vi "PH_Stepmotor_BaseClass.PC Write Axis PSDB.vi"(0 "i ref in":refnum<vi>, 5 "error IO":errorcluster) -> (14 "i ref out":refnum<vi>, 19 "error out":errorcluster)   [LabVIEW 2014, in "PH_Stepmotor_BaseClass.lvlib"]
doc: "This is the proc case which writes axis data to the PHELIX shot data base."
uses:
  PH_Stepmotor_BaseClass.lvlib
  PH_Stepmotor_BaseClass.Motor Type.ctl
  PH_PSDBWriter/PH_PSDBWriter.PSDB Dataset.ctl
  PH_PSDBWriter/PH_PSDBWriter.2D dataset.ctl
  CSlibraries-extern/psdb_lv/PSDB_AxisDescription.ctl
  PH_PSDBWriter/PH_PSDBWriter.Boolean dataset.ctl
  PH_PSDBWriter/PH_PSDBWriter.Image dataset.ctl
  <vilib>/vision/Image Controls.llb/IMAQ Image.ctl
  PH_PSDBWriter/PH_PSDBWriter.Numeric dataset.ctl
  PH_PSDBWriter/PH_PSDBWriter.String dataset.ctl
  PH_PSDBWriter/PH_PSDBWriter.Data Status.ctl
  PH_PSDBWriter/PH_PSDBWriter.lvlib
  CS_Core/CSSystem/CSSystemLib/CSSystemLib.lvlib
  CSlibraries-extern/psdb_lv/PSDB.lvlib
panel:
  in  "SW Scale.Motor Type":T1
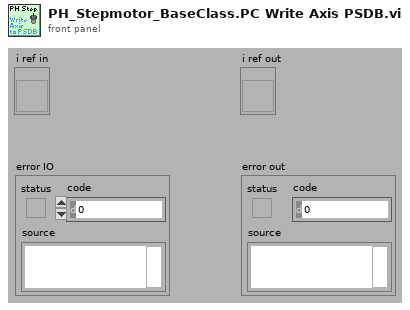
[diagram p1: front panel]
types:
  T1 = typedef "PH_Stepmotor_BaseClass.lvlib/PH_Stepmotor_BaseClass.Motor Type.ctl" = enum16{"Unspecific", "OWIS 49.120.2633", "OWIS 49.060.1033", "OWIS 43.040.2558", "Diamond Motion 2200 series", "OWIS 49.120.266B.MV6", "Calorimeter", "Linear Stage 1", "MICOS VT-80", "MICOS VT-80 S", "Standa Rotstage nt0.95A", "PUF RA 320.200", "PUF RA 800.200", "PUF RA 800.400", "PUF RA 400.50", "1324.nn.800.50", "1324.n9c.800.50", "1324.nn.320.200", "1324.nn.400.200", "1324.nn.800.200", "1324.nn.400.50", "1324.8c9c.800.50", "1324.8c9c.400.200"}
  T2 = typedef "PH_PSDBWriter.lvlib/PH_PSDBWriter.PSDB Dataset.ctl" = cluster{"Version":i32, "2D data Input":T3[], "Boolean Input":T5[], "Image Input":T6[], "Numeric Input":T8[], "String Input":T9[]}
  T3 = typedef "PH_PSDBWriter.lvlib/PH_PSDBWriter.2D dataset.ctl" = cluster{"name":string, "data":dbl[][], "axis description":T4}
  T4 = typedef "PSDB.lvlib/PSDB_AxisDescription.ctl" = cluster{"x axis label":string, "y axis label":string, "x axis unit":string, "y axis unit":string}
  T5 = typedef "PH_PSDBWriter.lvlib/PH_PSDBWriter.Boolean dataset.ctl" = cluster{"name":string, "data":bool, "unit":string}
  T6 = typedef "PH_PSDBWriter.lvlib/PH_PSDBWriter.Image dataset.ctl" = cluster{"name":string, "data":T7, "unit":string}
  T7 = typedef "IMAQ Image.ctl" = refnum<image>
  T8 = typedef "PH_PSDBWriter.lvlib/PH_PSDBWriter.Numeric dataset.ctl" = cluster{"name":string, "data":dbl, "unit":string}
  T9 = typedef "PH_PSDBWriter.lvlib/PH_PSDBWriter.String dataset.ctl" = cluster{"name":string, "data":string, "unit":string}
  T10 = typedef "PH_Stepmotor_BaseClass.lvlib/PH_Stepmotor_BaseClass.i attribute.ctl" = cluster{"Device Error":errorcluster, "Axes PSDB Thread":cluster{"Ref":refnum<vi>, "Q-Ref":refnum<queue>, "Data Status":T11}, "Axes":T12[], "Axes PSDB Infos":cluster{"GUI Name":string, "PSDB Instance ID":i32, "PSDB Status Service ID":i32, "Axis":i32, "Class":string}[], "GUI Refs":T16}
  T11 = typedef "PH_PSDBWriter.lvlib/PH_PSDBWriter.Data Status.ctl" = i16
  T12 = typedef "PH_Stepmotor_BaseClass.lvlib/PH_Stepmotor_BaseClass.Axis Attributes.ctl" = cluster{"Settings":T13, "Endswitch?":bool, "DIM Service IDs":T14, "Activity":T15, "Configured?":bool, "Position":cluster{"Current":i32, "Target":i32}, "Position to set":cluster{"New?":bool, "Wanted":i32}, "Stop?":bool, "Reset?":bool, "Move?":bool, "Nothing connected?":bool}
  T13 = typedef "PH_Stepmotor_BaseClass.lvlib/PH_Stepmotor_BaseClass.Axis Settings.ctl" = cluster{"Sign change":bool, "Width":dbl, "Calibration":dbl, "Unit":string, "Motor Type":T1, "Unit Width":string, "Unit CF":string}
  T14 = typedef "PH_Stepmotor_BaseClass.lvlib/PH_Stepmotor_BaseClass.Axis DIM Service IDs.ctl" = cluster{"Settings":i32, "Information":i32}
  T15 = typedef "PH_Stepmotor_BaseClass.lvlib/PH_Stepmotor_BaseClass.Axis Activity.ctl" = enum16{"No Information", "stopped", "running", "Failure", "Alarm", "stopped at backward ES", "stopped at foreward ES"}
  T16 = typedef "PH_Stepmotor_BaseClass.lvlib/PH_Stepmotor_BaseClass.GUI Refs.ctl" = cluster{"Axes Configuration":refnum<vi>, "Device Error":refnum<vi>, "Axes PSDB Infos":refnum<vi>}
  T17 = cluster{"GUI Name":string, "PSDB Instance ID":i32, "PSDB Status Service ID":i32, "Axis":i32, "Class":string}[]
  T18 = typedef "PH_PSDBWriter.lvlib/PH_PSDBWriter.i attribute.ctl" = cluster{"PSDB Status Service ID":i32, "Instance ID":i32, "Shot #":i32, "Subsystem":T19, "Data Status":T11, "Ref PSDB Status":refnum<vi>, "PSDB Error Code":i32, "PSDB Dataset":T2, "PSDB Thread":cluster{"Ref":refnum<vi>, "Q-Ref":refnum<queue>}, "PSDB Credentials":T20}
  T19 = typedef "PH_PSDBWriter.lvlib/PH_PSDBWriter.PHELIX-Subsystems.ctl" = i32
  T20 = typedef "PH_Common.lvlib/PH_Connection.PSDB Credentials.ctl" = cluster{"PW":string, "ID":string, "DS":string}
  T21 = cluster{"PSDB Instance ID":i32, "PSDB Dataset":T2}
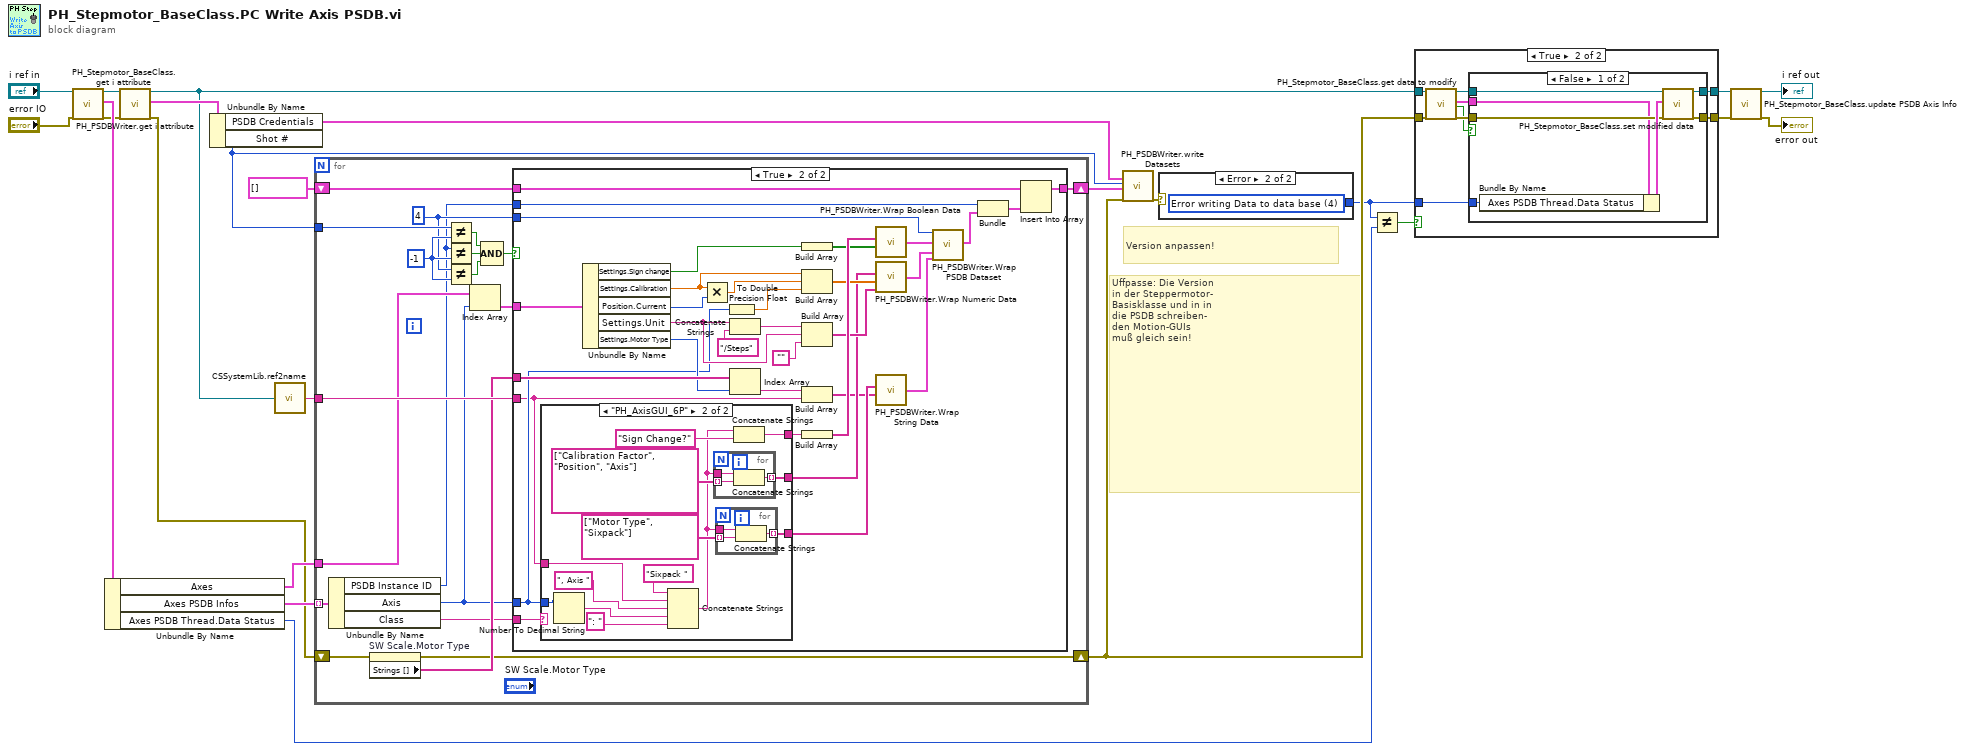
[diagram p0: block diagram]
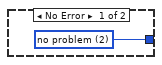
[diagram p4: hidden frame]
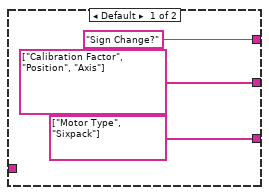
[diagram p6: hidden frame]
diagram:
  # "Uffpasse: Die Version\nin der Steppermotor-\nBasisklasse und in in\ndie PSDB schreiben-\nden Motion-GUIs\nmuß gleich sein!"
  # "Version anpassen!"
  n1 = call "PH_Stepmotor_BaseClass.get i attribute.vi"("i ref in"="i ref in", "error in (no error)"="error IO") -> ("i ref out"=w11:refnum<vi>, "i attribute"=w12:T10, "error out"=w9:errorcluster)  [unwired: 15 in]
  n2 = Unbundle By Name(w12) -> ("Axes"=w19:T12[], "Axes PSDB Infos"=w20:T17, "Axes PSDB Thread.Data Status"=w4:T11)
  n3 = call "PH_PSDBWriter.get i attribute.vi"("i ref in"=w11, "error in (no error)"=w9) -> ("i ref out"=w6:refnum<vi>, "i attribute"=w13:T18, "error out"=w5:errorcluster)  [unwired: 15 in]
  n4 = Unbundle By Name(w13) -> ("PSDB Credentials"=w1:T20, "Shot #"=w14:i32)
  n5 = call "CSSystemLib.ref2name.vi"("obj refnum"=w6) -> ("name"=w18:string)
  n6 = for {
    tunnel: w20 -> [w28] mode=indexing
    tunnel: w19 -> [w35]
    tunnel: w18 -> [w43]
    shift-right: [w32] -> w8
    shift-left: w5 -> [w33]
    tunnel: w14 -> [w40]
    shift-right: [w27] -> w15
    shift-left: cluster{"Version":i32, "PSDB Dataset":T2}[] [] ("Array") -> [w26]
    w29 = 4 ("Version")
    w42 = -1 ("y")
    n7 = Unbundle By Name(w28) -> ("PSDB Instance ID"=w25:i32, "Axis"=w30:i32, "Class"=w31:string)
    n8 = property on="SW Scale.Motor Type" class="Enum (strict)"(error in=w33) -> (error out=w32:errorcluster, "Strings []"=w36:string[])  [unwired: 1 in, 1 out]
    n9 = Not Equal?(x=w40, y=w42) -> (x != y?=w41:bool)
    n10 = Not Equal?(x=w25, y=w42) -> (x != y?=w39:bool)
    n11 = Not Equal?(x=w29, y=w42) -> (x != y?=w38:bool)
    n12 = Index Array(array=w35, index=w30) -> (element=w34:T12)
    n13 = Compound Arithmetic op=AND(w41, w39, w38) -> (w37:bool)
    n14 = case shown="True" w37 {
      tunnel: w36 -> [_ w77]
      tunnel: w43 -> [_ w66]
      tunnel: w29 -> [_ w49]
      tunnel: w34 -> [_ w71]
      tunnel: w31 -> [_ w69]
      tunnel: w30 -> [_ w67]
      tunnel: [w44 w47] -> w27
      tunnel: w26 -> [w44 w46]
      tunnel: w25 -> [_ w45]
      frame False {
      }
      frame True {
        n15 = case shown="\"PH_AxisGUI_6P\"" w69 {
          tunnel: w67 -> [_ w92]
          tunnel: [string[] ["Calibration Factor", "Position", "Axis"] w89] -> w56
          tunnel: ["Sign Change?" w88] -> w62
          tunnel: [string[] ["Motor Type", "Sixpack"] w84] -> w55
          tunnel: w66 -> [_ w82]
          frame Default {
          }
          frame "PH_AxisGUI_6P" {
            n16 = Number To Decimal String(number=w92) -> (decimal integer string=w91:string)  [unwired: 1 in]
            n17 = Concatenate Strings("Sixpack " ("string"), w82, ", Axis ", w91, ": " ("string")) -> (w85:string)
            n18 = for {
              tunnel: [w99] -> w89 mode=indexing
              tunnel: string[] ["Calibration Factor", "Position", "Axis"] -> [w98] mode=indexing
              tunnel: w85 -> [w97]
              n19 = Concatenate Strings(w97, w98) -> (w99:string)
            }
            n20 = for {
              tunnel: [w96] -> w84 mode=indexing
              tunnel: string[] ["Motor Type", "Sixpack"] -> [w95] mode=indexing
              tunnel: w85 -> [w94]
              n21 = Concatenate Strings(w94, w95) -> (w96:string)
            }
            n22 = Concatenate Strings(w85, "Sign Change?") -> (w88:string)
          }
        }
        n23 = Unbundle By Name(w71) -> ("Settings.Sign change"=w60:bool, "Settings.Calibration"=w65:dbl, "Position.Current"=w64:i32, "Settings.Unit"=w72:string, "Settings.Motor Type"=w76:T1)
        n24 = Multiply(x=w65, y=w64) -> (x*y=w63:dbl)
        n25 = To Double Precision Float(number=w67) -> (double precision float=w68:dbl)
        n26 = Concatenate Strings(w72, "/Steps" ("string")) -> (w74:string)
        n27 = Index Array(array=w77, index=w76) -> (element=w73:string)
        n28 = Build Array(w60) -> (w59:bool[])
        n29 = Build Array(w65, w63, w68) -> (w57:dbl[])
        n30 = Build Array(w74, w72, "" ("element")) -> (w58:string[])
        n31 = Build Array(w73, w66) -> (w54:string[])
        n32 = Build Array(w62) -> (w61:string[])
        n33 = call "PH_PSDBWriter.Wrap Boolean Data.vi"("Data Array"=w59, "Name Array"=w61) -> ("PSDB Boolean Data Array"=w53:T5[])  [unwired: 2 in]
        n34 = call "PH_PSDBWriter.Wrap Numeric Data.vi"("Unit Array"=w58, "Data Array"=w57, "Name Array"=w56) -> ("PSDB Numeric Data Array"=w52:T8[])  [unwired: 1 in]
        n35 = call "PH_PSDBWriter.Wrap String Data.vi"("Data Array"=w54, "Name Array"=w55) -> ("PSDB String Data Array"=w51:T9[])  [unwired: 2 in]
        n36 = call "PH_PSDBWriter.Wrap PSDB Dataset.vi"("Version"=w49, "Boolean Input"=w53, "Numeric Input"=w52, "String Input"=w51) -> ("PSDB Dataset"=w50:T2)  [unwired: 15 in]
        n37 = Bundle("PSDB Instance ID"=w45, "PSDB Dataset"=w50) -> (w48:T21)  [unwired: 1 in]
        n38 = Insert Into Array(array=w46, new element=w48) -> (w47:cluster{"Version":i32, "PSDB Dataset":T2}[])  [unwired: 1 in]
      }
    }
  }
  n39 = call "PH_PSDBWriter.write Datasets.vi"("PSDB Credentials"=w1, "Shot #"=w14, "Datasets"=w15, "error in (no error)"=w8) -> ("error out"=w17:errorcluster)  [unwired: 15 in]
  n40 = case shown="Error" w17 {
    tunnel: [w100 w101] -> w3
    frame No Error {
      w100 = T11 2 items=["no info", "no Data collection", "no problem", "Error getting the instance ID", "Error writing Data to data base", "Error concerning the subsystem"] ("Data Status")
    }
    frame Error {
      w101 = T11 4 items=["no info", "no Data collection", "no problem", "Error getting the instance ID", "Error writing Data to data base", "Error concerning the subsystem"] ("Data Status")
    }
  }
  n41 = Not Equal?(x=w3, y=w4) -> (x != y?=w2:bool)
  n42 = case shown="True" w2 {
    tunnel: [w103 w112] -> w23
    tunnel: [w102 w111] -> w21
    tunnel: w8 -> [w102 w106]
    tunnel: w6 -> [w103 w105]
    tunnel: w3 -> [_ w104]
    frame False {
    }
    frame True {
      n43 = call "PH_Stepmotor_BaseClass.get data to modify.vi"("i ref in"=w105, "error in (no error)"=w106) -> ("i ref out"=w110:refnum<vi>, "i attribute"=w108:T10, "timed out"=w107:bool, "error out"=w109:errorcluster)  [unwired: 14 in]
      n44 = case shown="False" w107 {
        tunnel: [w119 w121] -> w112
        tunnel: [w118 w120] -> w111
        tunnel: w110 -> [w116 w121]
        tunnel: w109 -> [w115 w120]
        tunnel: w108 -> [w114 _]
        tunnel: w104 -> [w113 _]
        frame False {
          n45 = Bundle By Name(cluster=w114, "Axes PSDB Thread.Data Status"=w113) -> (w117:T10)
          n46 = call "PH_Stepmotor_BaseClass.set modified data.vi"("i ref in"=w116, "i attribute"=w117, "error in (no error)"=w115) -> ("i ref out"=w119:refnum<vi>, "error out"=w118:errorcluster)  [unwired: 15 in]
        }
        frame True {
        }
      }
    }
  }
  n47 = call "PH_Stepmotor_BaseClass.update PSDB Axis Info.vi"("i ref in"=w23, "error in"=w21) -> ("i ref out"=→"i ref out":refnum<vi>, "error out"=→"error out":errorcluster)  [unwired: 16 in]
